vi "04_dosing.vi"() -> ()   [LabVIEW 2024]
uses:
  <vilib>/Utility/error.llb/DialogType.ctl
  <vilib>/DAQmx/miscellaneous.llb/DAQmx Fill In Error Info.vi
  <vilib>/Waveform/WDTOps.llb/WDT Waveform to XY Pairs DBL.vi
  <instrlib>/Tektronix DMM40x0 Series/Tektronix DMM40x0 Series.lvlib
panel:
  in  "error in":errorcluster
  out "Waveform Graph 2":dbl[](array[numeric])
  out "error out":errorcluster
  out "STABLE":bool
  in  "Serial Communication":T1={"Baud Rate"=9600, "Parity"=0, "Data Bits"=8, "Stop Bits"=10, "Flow Control"=0} {"Flow Control" items=["None", "XON/XOFF", "RTS/CTS", "XON/XOFF & RTS/CTS", "DTR/DSR", "XON/XOFF & DTR/DSR"]; "Stop Bits" items=["1.0"=10, "1.5"=15, "2.0"=20]; "Data Bits" items=["7"=7, "8"=8]; "Parity" items=["None", "Odd", "Even", "Mark", "Space"]; "Baud Rate" items=["300"=300, "600"=600, "1200"=1200, "2400"=2400, "4800"=4800, "9600"=9600, "19200"=19200]}
  in  "COM PORT (COM2)":refnum<visa-resource-name>
  out "Stability threshold":dbl format="%#_13g"
  out "Waveform Graph":dbl[](graph)
  out "XY pairs":cluster{"x":timestamp, "y":dbl}[](array[cluster]) {"y" format="%0.2f"}
  # "Voltmeter Serial Configuration"
  # "DEFAULT SETTINGS:\n\nTimeout (10000 ms)\nTrigger Count (5000)\nSample Count (1)\n\n****DC VOLTAGE***"
  # "Voltmeter Stability"
  # "0 - Stability threshold not met\n1 - Stability threshold met\n\n\n\n*stability (+/-0.05 mV) of last 15 pts"
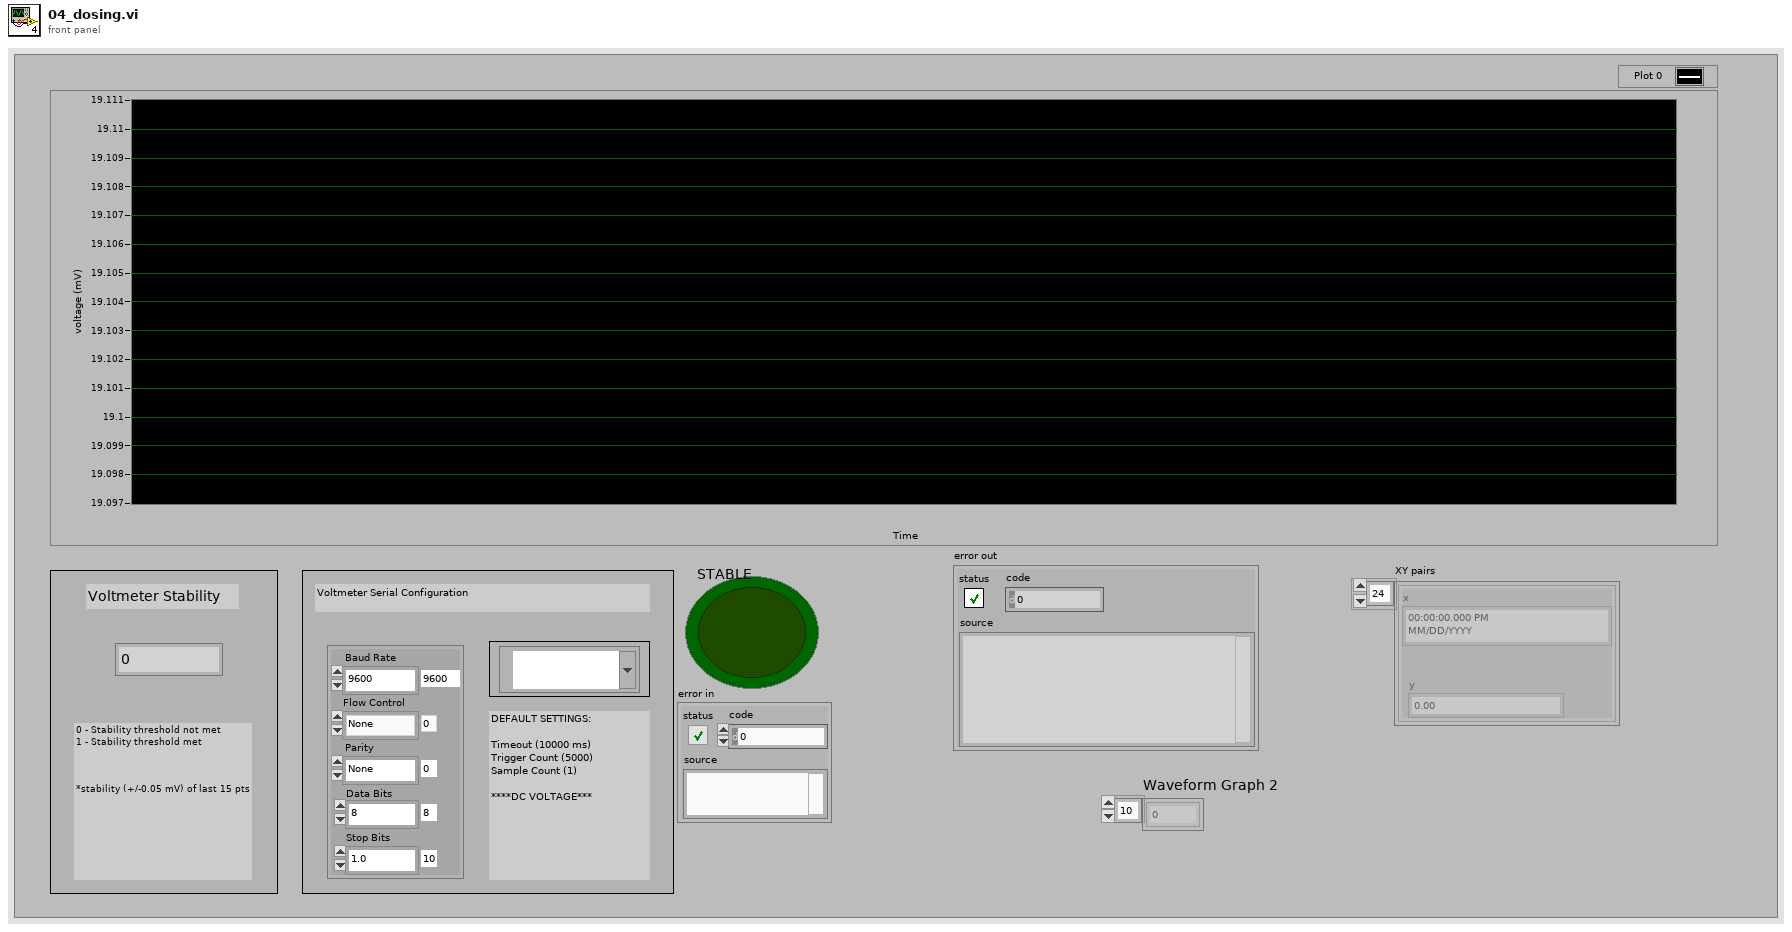
[diagram p1: front panel]
types:
  T1 = cluster{"Baud Rate":u32, "Parity":u16, "Data Bits":u16, "Stop Bits":u16, "Flow Control":u16}
  T2 = typedef "DialogType.ctl" = u16
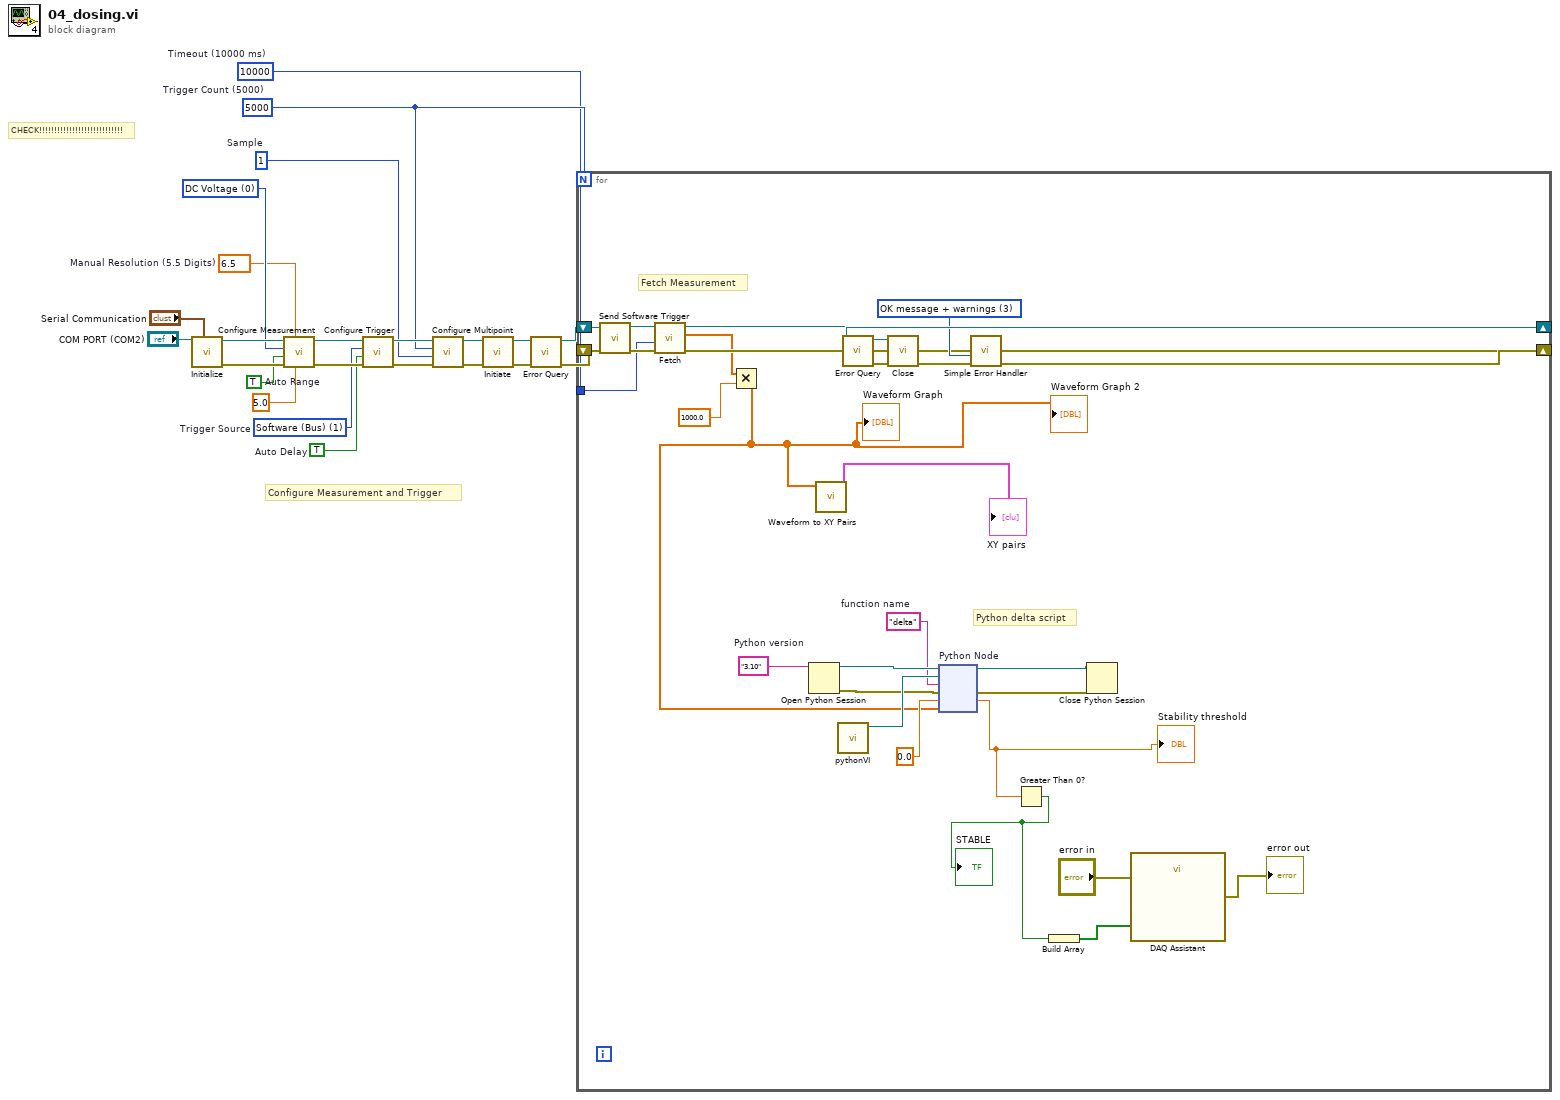
[diagram p0: block diagram]
diagram:
  w10 = u16 0 items=["DC Voltage", "AC Voltage", "2 - Wire Resistance", "4 - Wire Resistance", "DC Current", "AC Current", "Frequency", "Period", "Continuity", "Diode Checking", "Temperature", "Capacitance"] ("Function (0: DC Voltage)")
  w1 = u32 10000  # Timeout (10000 ms)
  w2 = 1  # Sample
  w9 = 5000  # Trigger Count (5000)
  w3 = 6.5 items=["4.5"=4.5, "5.5"=5.5, "6.5"=6.5]  # Manual Resolution (5.5 Digits)
  w11 = TRUE  # Auto Delay
  w12 = u16 1 items=["Immediate", "Software (Bus)", "External"]  # Trigger Source
  w13 = TRUE  # Auto Range
  w16 = T2 3 items=["no dialog", "OK message", "continue or stop message", "OK message + warnings", "continue/stop + warnings"] ("type of dialog (OK msg:1)")
  # "CHECK!!!!!!!!!!!!!!!!!!!!!!!!!!!!"
  # "Configure Measurement and Trigger"
  n1 = call <instrlib>:"Initialize.vi"("Serial Configuration"="Serial Communication", "VISA resource name"="COM PORT (COM2)") -> ("error out"=w28:errorcluster, "VISA resource name out"=w29:refnum<visa-resource-name>)  [unwired: 3 in, 5 out]
  n2 = call <instrlib>:"Configure Measurement.vi"("Manual Range (1.0)"=5.0, "Manual Resolution (5.5 Digits)"=w3, "error in (no error)"=w28, "Auto Range (T:Enable)"=w13, "Function (0: DC Voltage)"=w10, "VISA resource name"=w29) -> ("error out"=w26:errorcluster, "VISA resource name out"=w27:refnum<visa-resource-name>)  [unwired: 4 out]
  n3 = call <instrlib>:"Configure Trigger.vi"("error in (no error)"=w26, "Auto Delay (T: Enable)"=w11, "Trigger Source (0: Immediate)"=w12, "VISA resource name"=w27) -> ("error out"=w24:errorcluster, "VISA resource name out"=w25:refnum<visa-resource-name>)  [unwired: 1 in, 5 out]
  n4 = call <instrlib>:"Configure Multipoint.vi"("error in (no error)"=w24, "Sample Count (1)"=w2, "Trigger Count (1)"=w9, "VISA resource name"=w25) -> ("error out"=w21:errorcluster, "VISA resource name out"=w22:refnum<visa-resource-name>)  [unwired: 6 out]
  n5 = call <instrlib>:"Initiate.vi"("error in (no error)"=w21, "VISA resource name"=w22) -> ("error out"=w8:errorcluster, "VISA resource name out"=w7:refnum<visa-resource-name>)  [unwired: 8 out]
  n6 = call <instrlib>:"Error Query.vi"("error in (no error)"=w8, "VISA resource name"=w7) -> ("error out"=w5:errorcluster, "VISA resource name out"=w6:refnum<visa-resource-name>)  [unwired: 8 out]
  n7 = for {
    N: w9 -> [_]
    shift-right: [w52] -> w18
    shift-left: w5 -> [w48]
    shift-right: [w53] -> w20
    shift-left: w6 -> [w49]
    tunnel: w1 -> [w47]
    w39 = "delta"  # function name
    w37 = "3.10"  # Python version
    # "Python delta script"
    # "Fetch Measurement"
    n8 = call <instrlib>:"Send Software Trigger.vi"("error in (no error)"=w48, "VISA resource name"=w49) -> ("error out"=w50:errorcluster, "VISA resource name out"=w51:refnum<visa-resource-name>)  [unwired: 8 out]
    n9 = call <instrlib>:"Fetch.vi"("error in (no error)"=w50, "Timeout (10000 ms)"=w47, "VISA resource name"=w51) -> ("error out"=w52:errorcluster, "Measurements"=w46:dbl[], "VISA resource name out"=w53:refnum<visa-resource-name>)  [unwired: 6 out]
    n10 = Multiply(x=w46, y=1000.0) -> (x*y=w33:dbl[])
    "Waveform Graph" <- w33
    "Waveform Graph 2" <- w33
    n11 = Open Python Session(python version=w37) -> (session out=w43:refnum<k35>, error out=w40:errorcluster)  [unwired: 2 in]
    n12 = call-poly <vilib>:"Waveform to XY Pairs.vi"("waveform in"=w33) -> ("XY pairs"=→"XY pairs":cluster{"x":timestamp, "y":dbl}[])  [unwired: 8 in, 2 out]
    n13 = call "pythonVI.vi"() -> ("appended path"=w44:path)  [unwired: 11 in]
    n14 = node "Python Node"(w43, w44, w39, w40, 0.0, w33) -> (w42:refnum<k35>, w41:errorcluster, w36:dbl)  [unwired: 1 in, 2 out]
    "Stability threshold" <- w36
    n15 = Greater Than 0?(x=w36) -> (x > 0?=w31:bool)
    "STABLE" <- w31
    n16 = Build Array(w31) -> (w34:bool[])
    n17 = Close Python Session(session in=w42, error in=w41) -> ()  [unwired: 1 out]
    n18 = call "DAQ Assistant"("data"=w34, "error in"="error in") -> ("error out"=→"error out":errorcluster)  [unwired: 16 in, 1 out]
  }
  n19 = call <instrlib>:"Error Query.vi"("error in (no error)"=w18, "VISA resource name"=w20) -> ("error out"=w17:errorcluster, "VISA resource name out"=w19:refnum<visa-resource-name>)  [unwired: 8 out]
  n20 = call <instrlib>:"Close.vi"("error in (no error)"=w17, "VISA resource name"=w19) -> ("error out"=w23:errorcluster)  [unwired: 9 out]
  n21 = call <vilib>:"Simple Error Handler.vi"("type of dialog (OK msg:1)"=w16, "error in (no error)"=w23) -> ()  [unwired: 8 out]
